vi "Search Closest Element In 1D Array.vi"(9 "Start index":i32, 10 "Desired element":dbl format="%#_13g", 11 "1D Array":dbl[](array[numeric])) -> (2 "Closest Index":i32, 3 "Closest Element":dbl)   [LabVIEW 2022 SP3, in "Decimation.lvlib"]
doc: "Find the closest elements from 1D array."
uses:
  Decimation.lvlib
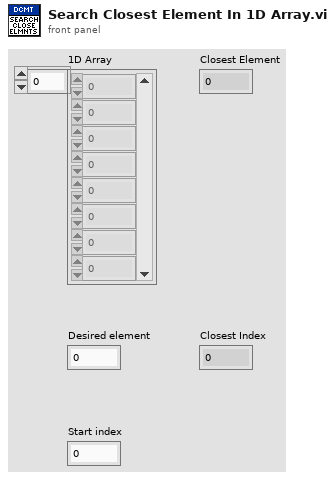
[diagram p1: front panel]
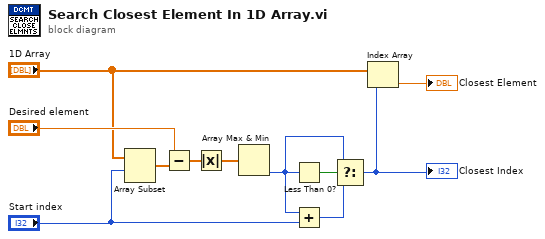
[diagram p0: block diagram]
diagram:
  n1 = Array Subset(array="1D Array", index="Start index") -> (w3:dbl[])  [unwired: 1 in]
  n2 = Subtract(x="Desired element", y=w3) -> (x-y=w5:dbl[])
  n3 = Absolute Value(x=w5) -> (abs(x)=w6:dbl[])
  n4 = Array Max & Min(array=w6) -> (min index (indices)=w10:i32)  [unwired: 3 out]
  n5 = Less Than 0?(x=w10) -> (x < 0?=w8:bool)
  n6 = Add(x=w10, y="Start index") -> (x+y=w9:i32)
  n7 = Select(t=w10, s=w8, f=w9) -> (s? t:f=w11:i32)
  "Closest Index" <- w11
  n8 = Index Array(array="1D Array", index=w11) -> (element=→"Closest Element":dbl)
